vi "HVBuncher.SetChannelVoltage.vi"(0 "i ref in":refnum<vi>, 1 "channel":i32, 2 "Voltage in V":dbl format="%.2f", 3 "ms timeout (10000)":i32=10000, 5 "error in (no error)":errorcluster) -> (14 "i ref out":refnum<vi>, 18 "timed out":bool, 19 "error out":errorcluster)   [LabVIEW 2014, in "HVBuncher.lvlib"]
doc: "Sets the voltage."
uses:
  HVBuncher.lvlib
  CSCore/CSApplicationBaseClasses/PSChannelBase/PSChannelBase.directionType.ctl
  CSCore/CSApplicationBaseClasses/PSChannelBase/PSChannelBase.serviceType.ctl
  CSlibraries/UtilityLib/UtilityLib.valueStatus.ctl
  CSCore/CSApplicationBaseClasses/PSChannelBase/PSChannelBase.lvlib
  CSlibraries/UtilityLib/UtilityLib.lvlib
  CSCore/CSApplicationBaseClasses/DeviceBase/DeviceBase.lvlib
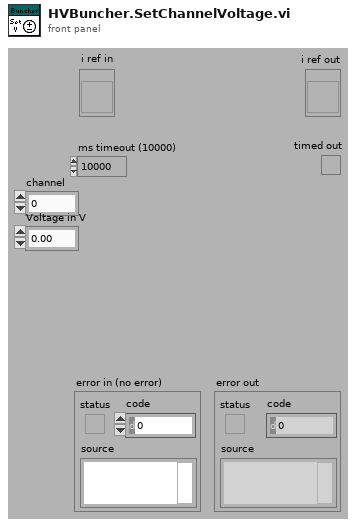
[diagram p1: front panel]
types:
  T1 = typedef "PSChannelBase.lvlib/PSChannelBase.directionType.ctl" = enum16{"unknown", "update actual value", "update nominal value", "update both"}
  T2 = typedef "PSChannelBase.lvlib/PSChannelBase.serviceType.ctl" = enum16{"onOff", "voltage", "current", "tripCurrent", "rampUpSpeed", "rampDownSpeed", "status"}
  T3 = typedef "UtilityLib.lvlib/UtilityLib.valueStatus.ctl" = enum16{"no info available", "stand by/off", "on", "warning", "alarm/malfunction", "not implemented", "user action required", "important information", "system default", "control default", "indicator default", "button default"}
  T4 = typedef "PSChannelBase.lvlib/PSChannelBase.i attribute.ctl" = cluster{"defaultChannelIndex":i32, "nofChannels":i32, "defaultChannelIndexID":i32, "nofChannelsID":i32, "actValues":T5, "nomValues":T5, "logicalName":string[], "physicalName":string[], "logicalNameID":i32, "physicalNameID":i32}
  T5 = typedef "PSChannelBase.lvlib/PSChannelBase.parameters.ctl" = cluster{"onOff":bool[], "voltage":dbl[], "current":dbl[], "tripCurrent":dbl[], "rampUpSpeed":dbl[], "rampDownSpeed":dbl[], "status":i32[], "serviceIDs":cluster{"onOfflID":i32, "voltageID":i32, "currentID":i32, "tripCurrentID":i32, "rampUpSpeedID":i32, "rampDownSpeedID":i32, "statusID":i32}}
  T6 = typedef "HVBuncher.lvlib/HVBuncher.i attribute.ctl" = cluster{"ObjectsInitialized":bool, "ChildObjects":T7}
  T7 = typedef "HVBuncher.lvlib/HVBuncher.ChildObjects.ctl" = cluster{"ObjectsLoaded":string[], "actVoltage":dbl[]}
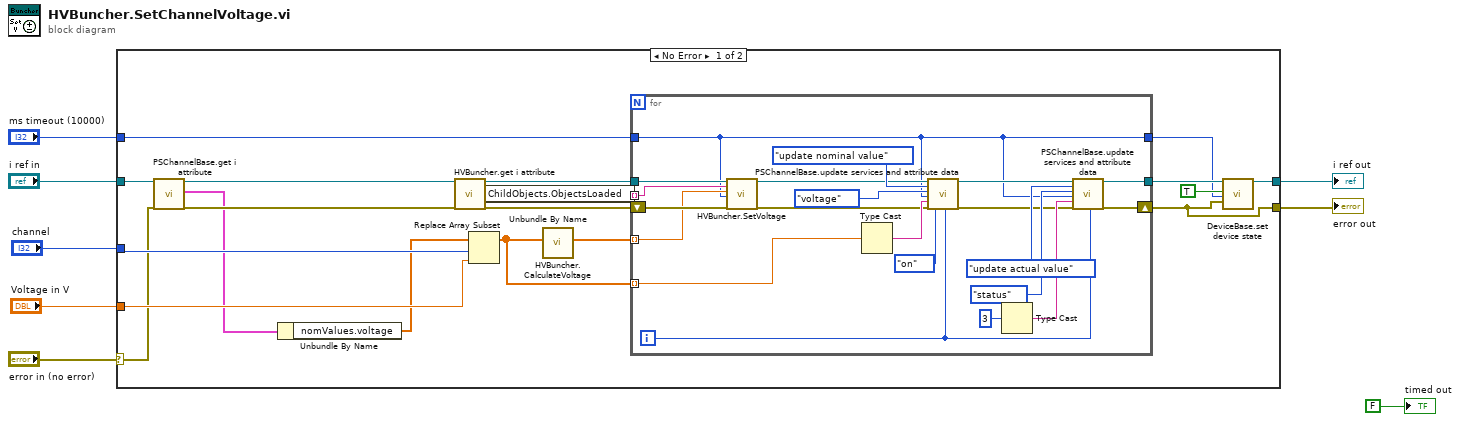
[diagram p0: block diagram]
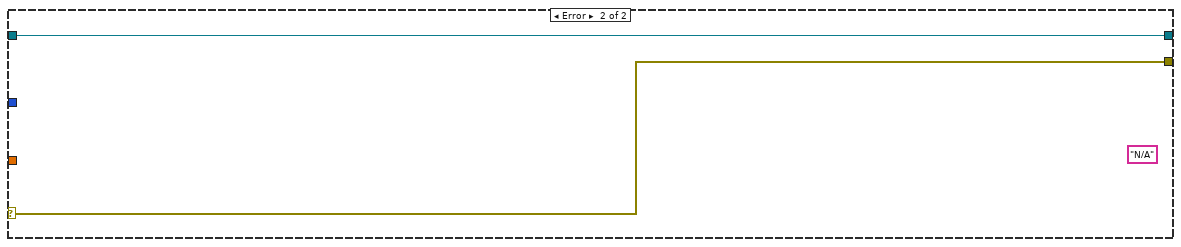
[diagram p2: hidden frame]
diagram:
  n1 = case shown="No Error" "error in (no error)" {
    selector: "error in (no error)" -> [w22 w50]
    tunnel: "i ref in" -> [w28 w51]
    tunnel: [w11 w51] -> w7
    tunnel: [w9 w50] -> w5
    tunnel: "ms timeout (10000)" -> [w15 _]
    tunnel: "channel" -> [w27 _]
    tunnel: "Voltage in V" -> [w26 _]
    frame No Error {
      n2 = call "PSChannelBase.get i attribute.vi"("i ref in"=w28, "error in (no error)"=w22) -> ("i ref out"=w25:refnum<vi>, "i attribute"=w17:T4, "error out"=w21:errorcluster)  [unwired: 15 in]
      n3 = Unbundle By Name(w17) -> ("nomValues.voltage"=w19:dbl[])
      n4 = call "HVBuncher.get i attribute.vi"("i ref in"=w25, "error in (no error)"=w21) -> ("i ref out"=w23:refnum<vi>, "i attribute"=w24:T6, "error out"=w18:errorcluster)  [unwired: 15 in]
      n5 = Unbundle By Name(w24) -> ("ChildObjects.ObjectsLoaded"=w20:string[])
      n6 = Replace Array Subset(array=w19, new element=w26, index=w27) -> (w14:dbl[])
      n7 = call "HVBuncher.CalculateVoltage.vi"("nomVoltages"=w14) -> ("ChannelVoltages"=w16:dbl[])  [unwired: 10 in]
      n8 = for {
        tunnel: w23 -> [w49]
        tunnel: w15 -> [w29]
        tunnel: w16 -> [w40] mode=indexing
        tunnel: w20 -> [w48] mode=indexing
        shift-right: [w33] -> w9
        shift-left: w18 -> [w47]
        tunnel: w14 -> [w39] mode=indexing
        tunnel: [w34] -> w12
        tunnel: [w29] -> w10
        i -> [w31]
        n9 = call "HVBuncher.SetVoltage.vi"("i ref in"=w49, "Object"=w48, "SetVoltage"=w40, "ms timeout (10000)"=w29, "error in (no error)"=w47) -> ("i ref out"=w42:refnum<vi>, "error out"=w41:errorcluster)  [unwired: 12 in, 1 out]
        n10 = Type Cast(x=w39) -> (*(type *) &x=w44:string)  [unwired: 1 in]
        n11 = call "PSChannelBase.update services and attribute data.vi"("i ref in"=w42, "direction"=PSChannelBase.directionType."update nominal value", "service"=PSChannelBase.serviceType."voltage", "ms timeout (10000)"=w29, "value"=w44, "error in (no error)"=w41, "quality"=UtilityLib.valueStatus."on", "channelNumber"=w31) -> ("i ref out"=w35:refnum<vi>, "error out"=w32:errorcluster)  [unwired: 9 in, 1 out]
        n12 = Type Cast(x=3) -> (*(type *) &x=w36:string)  [unwired: 1 in]
        n13 = call "PSChannelBase.update services and attribute data.vi"("i ref in"=w35, "direction"=PSChannelBase.directionType."update actual value", "service"=PSChannelBase.serviceType."status", "ms timeout (10000)"=w29, "value"=w36, "error in (no error)"=w32, "channelNumber"=w31) -> ("i ref out"=w34:refnum<vi>, "error out"=w33:errorcluster)  [unwired: 10 in, 1 out]
      }
      n14 = call "DeviceBase.set device state.vi"("i ref in"=w12, "implicit"=TRUE, "ms timeout (10000)"=w10, "device error"=w9) -> ("i ref out"=w11:refnum<vi>)  [unwired: 13 in, 2 out]
    }
    frame Error {
      (unwired) "N/A"
    }
  }
  "error out" <- w5
  "i ref out" <- w7
  "timed out" <- FALSE ("timed out")
